vi "Facade 1.vi"(0 "Data In":T5, 2 "Display State In":T3, 3 "Container State":T4) -> (6 "Data Out":T5, 7 "Display State Out":T3, 8 "Action":T2)   [LabVIEW 2015, in "ECS-Host.lvlib" / "TrackingChart.xctl"]
uses:
  TrackingChart.xctl
  Data 1.ctl
  <vilib>/_xctls/Container State.ctl
  State 1.ctl
  <vilib>/_xctls/Action.ctl
  <vilib>/_xctls/XControlSupport.lvlib
panel:
  out "Chart":T1(graph)
  out "Indicator 1":sgl(slide) scale=0.0..25.0 scale format="%#.1f"
  out "Indicator 2":sgl(slide) scale=0.0..25.0 scale format="%#.1f"
  out "Indicator 3":sgl(slide) scale=0.0..25.0 scale format="%#.1f"
  out "Indicator 4":sgl(slide) scale=0.0..25.0 scale format="%#.1f"
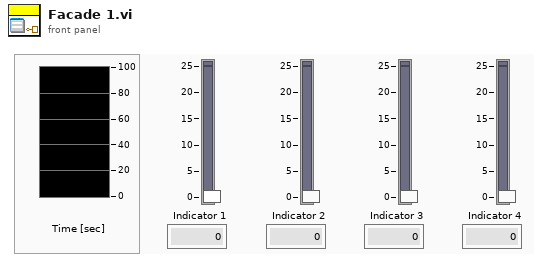
[diagram p1: front panel]
types:
  T1 = cluster{"[0]":sgl, "[1]":sgl, "[2]":sgl, "[3]":sgl, "[4]":sgl, "[5]":sgl, "[6]":sgl, "[7]":sgl, "[8]":sgl}
  T2 = typedef "XControlSupport.lvlib/Action.ctl" = cluster{"Data Changed?":bool, "State Changed?":bool, "Action Name":string}
  T3 = typedef "ECS-Host.lvlib/TrackingChart.xctl/State 1.ctl" = cluster{"Numeric":dbl}
  T4 = typedef "XControlSupport.lvlib/Container State.ctl" = cluster{"Indicator?":bool, "Run Mode?":bool, " Refnum":refnum<vi>}
  T5 = typedef "ECS-Host.lvlib/TrackingChart.xctl/Data 1.ctl" = cluster{"Value":sgl, "Name":string, "Unit":string, "Max":sgl, "Min":sgl}[]
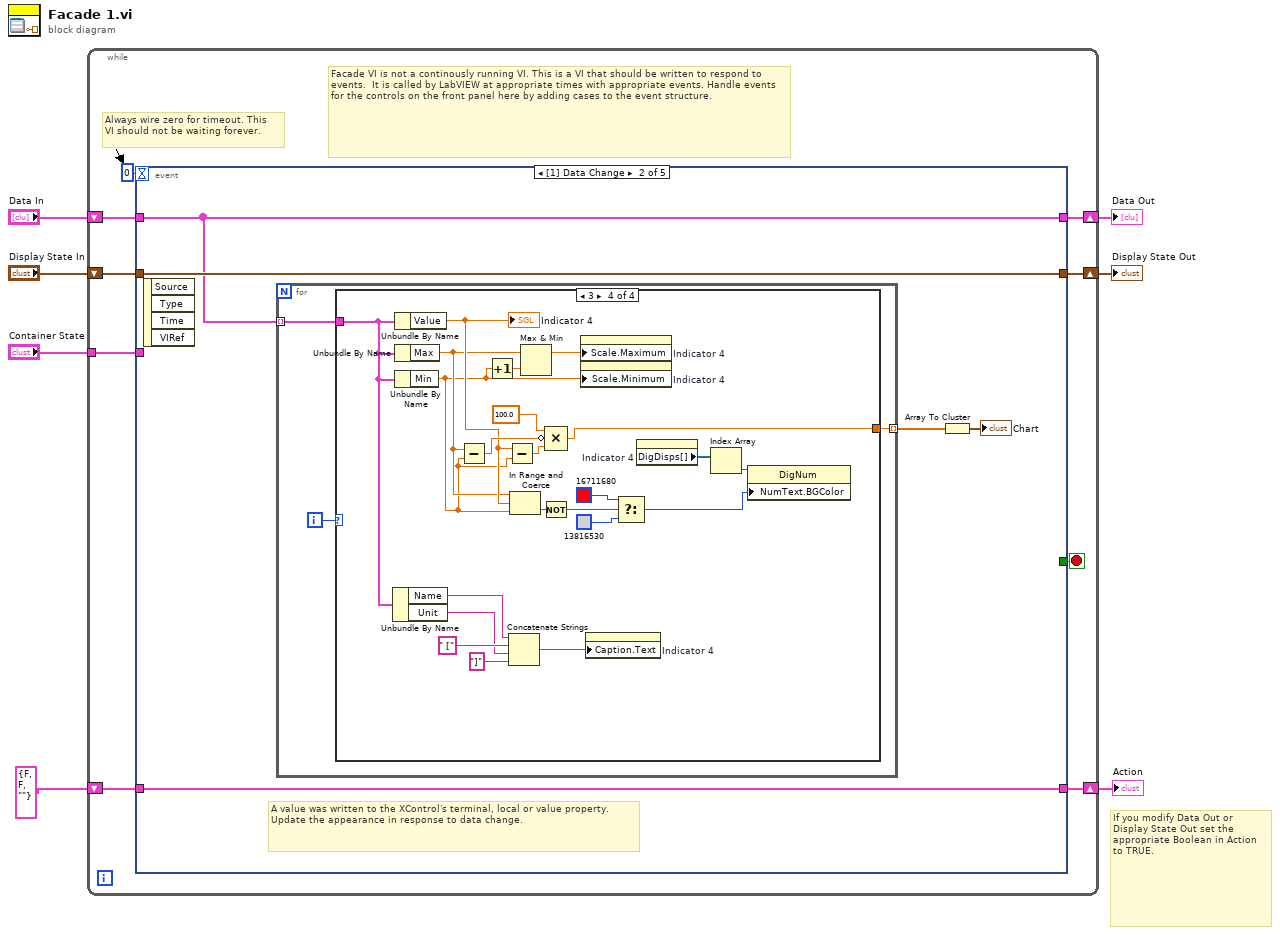
[diagram p0: block diagram]
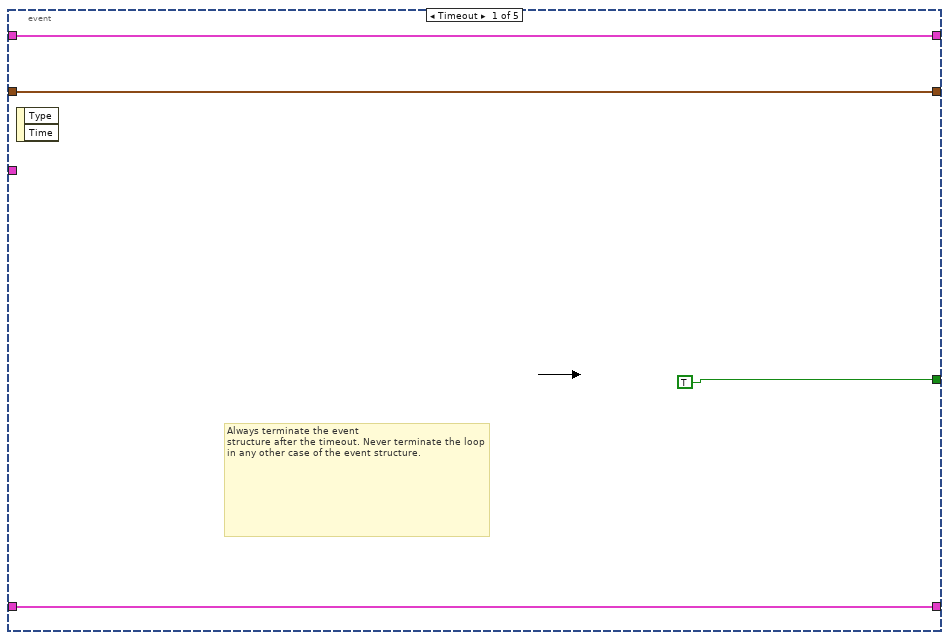
[diagram p2: hidden frame]
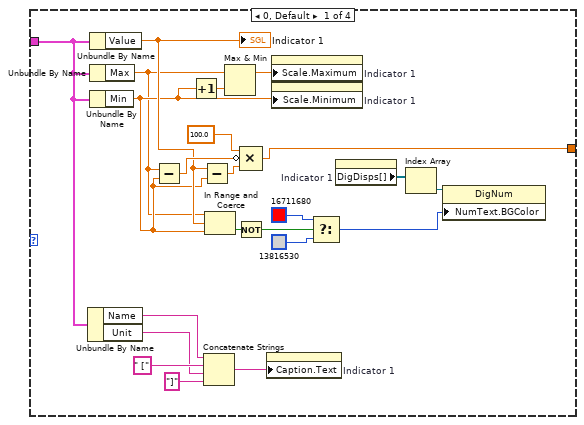
[diagram p3: hidden frame]
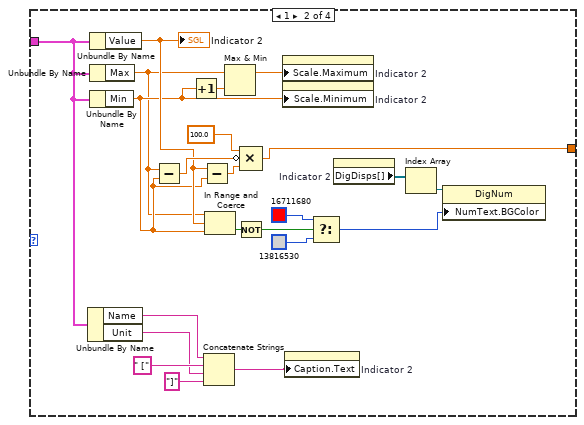
[diagram p4: hidden frame]
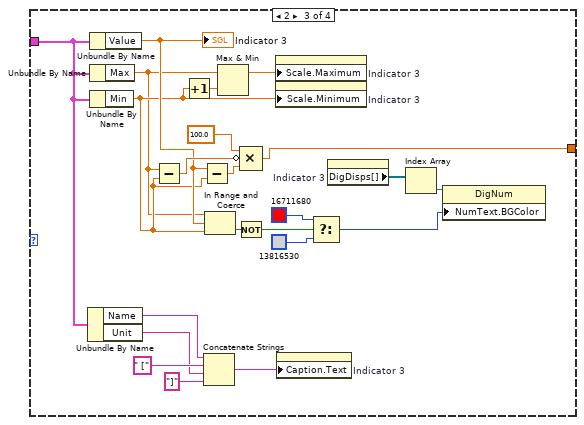
[diagram p5: hidden frame]
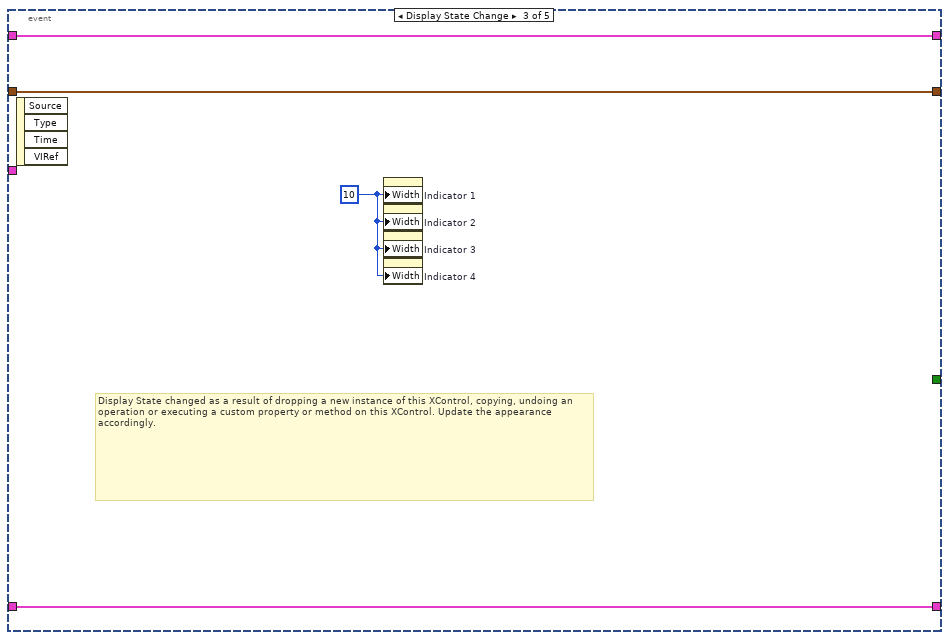
[diagram p6: hidden frame]
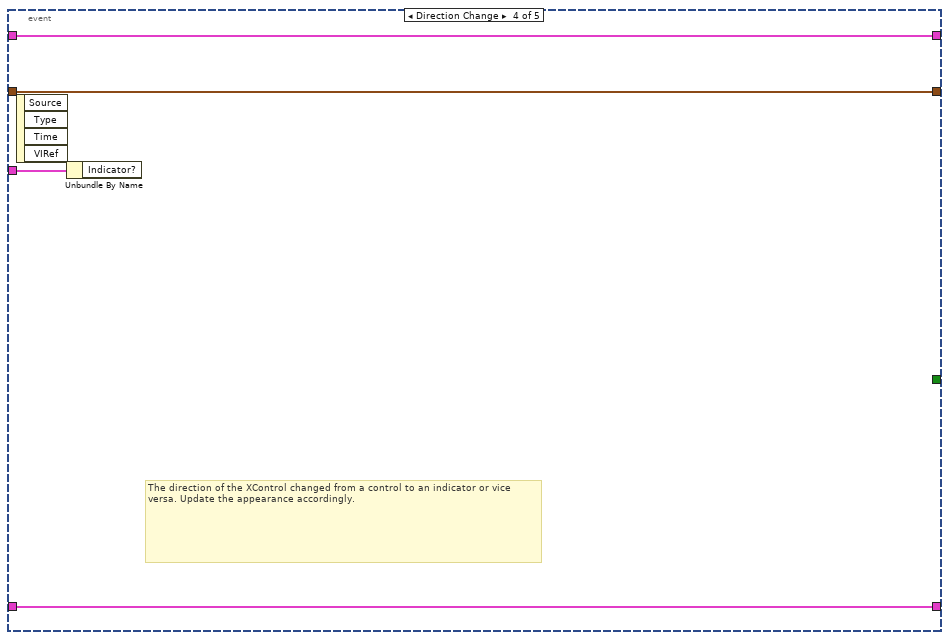
[diagram p7: hidden frame]
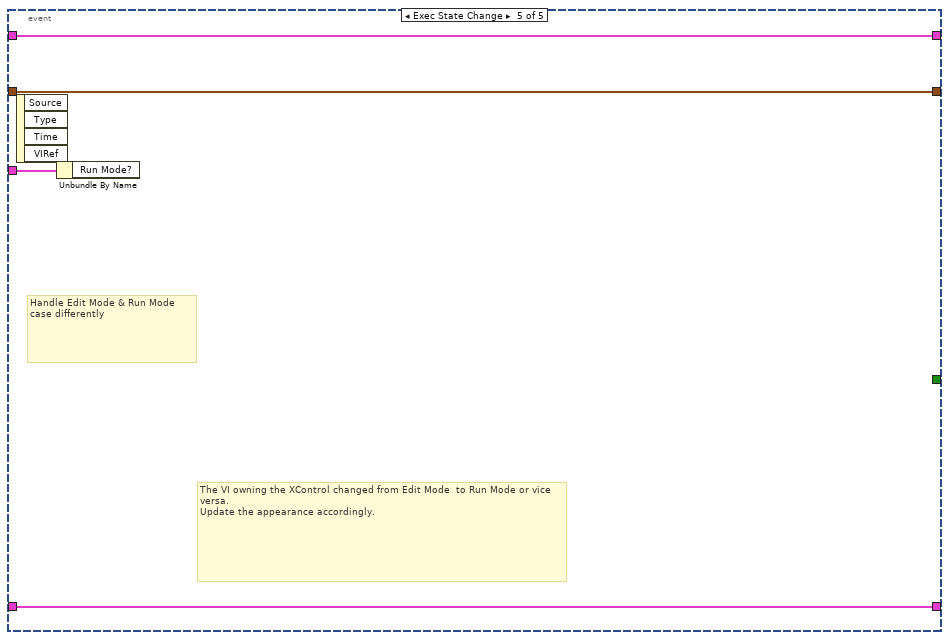
[diagram p8: hidden frame]
diagram:
  # "If you modify Data Out or\nDisplay State Out set the\nappropriate Boolean in Action\nto TRUE."
  n1 = while {
    shift-right: [w15] -> w4
    shift-left: "Display State In" -> [w16]
    tunnel: "Container State" -> [w12]
    shift-right: [w10] -> w7
    shift-left: "Data In" -> [w11]
    shift-right: [w8] -> w2
    shift-left: T2 {"Data Changed?"=FALSE, "State Changed?"=FALSE, "Action Name"=""} ("Action") -> [w9]
    stop <- w14 stop-if-true
    # "Facade VI is not a continously running VI. This is a VI that should be written to respond to events.  It is called by LabVIEW at appropriate times with appropriate events. Handle events for the controls on the front panel here by adding cases to the event structure."
    # "Always wire zero for timeout. This\nVI should not be waiting forever."
    n2 = event shown="[1] Data Change" {
      selector: _ -> [_ _ _ _ _]
      dyn-events: _ -> [_ _ _ _ _]
      timeout: 0 -> [_ _ _ _ _]
      tunnel: w16 -> [w18 w25 w120 w123 w127]
      tunnel: [w18 w25 w120 w123 w127] -> w15
      tunnel: [TRUE _ _ _ _] -> w14
      tunnel: w12 -> [_ _ _ w124 w128]
      tunnel: w11 -> [w17 w21 w118 w122 w125]
      tunnel: [w17 w21 w118 w122 w125] -> w10
      tunnel: [w19 w24 w119 w121 w126] -> w8
      tunnel: w9 -> [w19 w24 w119 w121 w126]
      event Timeout {
        # "Always terminate the event\nstructure after the timeout. Never terminate the loop in any other case of the event structure."
        n3 = event-data() -> ()  [unwired: 1 in, 2 out]
      }
      event Data Change {
        # "A value was written to the XControl's terminal, local or value property.\nUpdate the appearance in response to data change."
        n4 = event-data() -> ()  [unwired: 1 in, 4 out]
        n5 = for {
          tunnel: w21 -> [w27] mode=indexing
          tunnel: [w26] -> w22 mode=indexing
          i -> [w28]
          n6 = case shown="3" w28 {
            tunnel: w27 -> [w47 w69 w91 w113]
            tunnel: [w33 w58 w80 w102] -> w26
            frame 0, Default {
              n7 = Unbundle By Name(w47) -> ("Name"=w46:string, "Unit"=w48:string)
              n8 = Unbundle By Name(w47) -> ("Value"=w40:sgl)
              "Indicator 1" <- w40
              n9 = Unbundle By Name(w47) -> ("Max"=w29:sgl)
              n10 = Unbundle By Name(w47) -> ("Min"=w31:sgl)
              n11 = Subtract(x=w29, y=w31) -> (x-y=w42:sgl)
              n12 = Increment(x=w31) -> (x+1=w30:sgl)
              n13 = Subtract(x=w40, y=w31) -> (x-y=w44:sgl)
              n14 = Concatenate Strings(w46, " [", w48, "]") -> (w45:string)
              n15 = In Range and Coerce(upper limit=w29, x=w40, lower limit=w31) -> (In Range?=w41:bool)  [unwired: 1 out]
              n16 = Max & Min(x=w29, y=w30) -> (max(x,y)=w32:sgl)  [unwired: 1 out]
              n17 = Not(x=w41) -> (.not. x?=w37:bool)
              n18 = Compound Arithmetic op=MULTIPLY(sgl 100.0 ("value"), invert w42, w44) -> (w33:sgl)
              n19 = property on="Indicator 1" class="Slide (strict)"("Caption.Text"=w45) -> ()  [unwired: 2 in, 2 out]
              n20 = property on="Indicator 1" class="Slide (strict)"("Scale.Maximum"=w32) -> ()  [unwired: 2 in, 2 out]
              n21 = property on="Indicator 1" class="Slide (strict)"("Scale.Minimum"=w31) -> ()  [unwired: 2 in, 2 out]
              n22 = Select(t=u32 16711680, s=w37, f=u32 13816530) -> (s? t:f=w36:u32)
              n23 = property on="Indicator 1" class="Slide (strict)"() -> ("DigDisps[]"=w35:refnum<vi>[])  [unwired: 2 in, 2 out]
              n24 = Index Array(array=w35) -> (element=w34:refnum<vi>)  [unwired: 1 in]
              n25 = property class="DigNum"(reference=w34, "NumText.BGColor"=w36) -> ()  [unwired: 1 in, 2 out]
            }
            frame 1 {
              n26 = Unbundle By Name(w69) -> ("Name"=w68:string, "Unit"=w70:string)
              n27 = Unbundle By Name(w69) -> ("Value"=w55:sgl)
              "Indicator 2" <- w55
              n28 = Unbundle By Name(w69) -> ("Max"=w51:sgl)
              n29 = Unbundle By Name(w69) -> ("Min"=w53:sgl)
              n30 = Subtract(x=w51, y=w53) -> (x-y=w65:sgl)
              n31 = Increment(x=w53) -> (x+1=w54:sgl)
              n32 = Subtract(x=w55, y=w53) -> (x-y=w67:sgl)
              n33 = Concatenate Strings(w68, " [", w70, "]") -> (w57:string)
              n34 = In Range and Coerce(upper limit=w51, x=w55, lower limit=w53) -> (In Range?=w64:bool)  [unwired: 1 out]
              n35 = Max & Min(x=w51, y=w54) -> (max(x,y)=w52:sgl)  [unwired: 1 out]
              n36 = Not(x=w64) -> (.not. x?=w61:bool)
              n37 = Compound Arithmetic op=MULTIPLY(sgl 100.0 ("value"), invert w65, w67) -> (w58:sgl)
              n38 = property on="Indicator 2" class="Slide (strict)"("Scale.Maximum"=w52) -> ()  [unwired: 2 in, 2 out]
              n39 = property on="Indicator 2" class="Slide (strict)"("Scale.Minimum"=w53) -> ()  [unwired: 2 in, 2 out]
              n40 = property on="Indicator 2" class="Slide (strict)"("Caption.Text"=w57) -> ()  [unwired: 2 in, 2 out]
              n41 = Select(t=u32 16711680, s=w61, f=u32 13816530) -> (s? t:f=w60:u32)
              n42 = property on="Indicator 2" class="Slide (strict)"() -> ("DigDisps[]"=w56:refnum<vi>[])  [unwired: 2 in, 2 out]
              n43 = Index Array(array=w56) -> (element=w59:refnum<vi>)  [unwired: 1 in]
              n44 = property class="DigNum"(reference=w59, "NumText.BGColor"=w60) -> ()  [unwired: 1 in, 2 out]
            }
            frame 2 {
              n45 = Unbundle By Name(w91) -> ("Name"=w90:string, "Unit"=w92:string)
              n46 = Unbundle By Name(w91) -> ("Value"=w79:sgl)
              "Indicator 3" <- w79
              n47 = Unbundle By Name(w91) -> ("Max"=w73:sgl)
              n48 = Unbundle By Name(w91) -> ("Min"=w75:sgl)
              n49 = Subtract(x=w73, y=w75) -> (x-y=w87:sgl)
              n50 = Increment(x=w75) -> (x+1=w76:sgl)
              n51 = Subtract(x=w79, y=w75) -> (x-y=w89:sgl)
              n52 = Concatenate Strings(w90, " [", w92, "]") -> (w78:string)
              n53 = In Range and Coerce(upper limit=w73, x=w79, lower limit=w75) -> (In Range?=w86:bool)  [unwired: 1 out]
              n54 = Max & Min(x=w73, y=w76) -> (max(x,y)=w74:sgl)  [unwired: 1 out]
              n55 = Not(x=w86) -> (.not. x?=w83:bool)
              n56 = Compound Arithmetic op=MULTIPLY(sgl 100.0 ("value"), invert w87, w89) -> (w80:sgl)
              n57 = property on="Indicator 3" class="Slide (strict)"("Scale.Maximum"=w74) -> ()  [unwired: 2 in, 2 out]
              n58 = property on="Indicator 3" class="Slide (strict)"("Scale.Minimum"=w75) -> ()  [unwired: 2 in, 2 out]
              n59 = property on="Indicator 3" class="Slide (strict)"("Caption.Text"=w78) -> ()  [unwired: 2 in, 2 out]
              n60 = Select(t=u32 16711680, s=w83, f=u32 13816530) -> (s? t:f=w82:u32)
              n61 = property on="Indicator 3" class="Slide (strict)"() -> ("DigDisps[]"=w77:refnum<vi>[])  [unwired: 2 in, 2 out]
              n62 = Index Array(array=w77) -> (element=w81:refnum<vi>)  [unwired: 1 in]
              n63 = property class="DigNum"(reference=w81, "NumText.BGColor"=w82) -> ()  [unwired: 1 in, 2 out]
            }
            frame 3 {
              n64 = Unbundle By Name(w113) -> ("Name"=w112:string, "Unit"=w114:string)
              n65 = Unbundle By Name(w113) -> ("Value"=w100:sgl)
              "Indicator 4" <- w100
              n66 = Unbundle By Name(w113) -> ("Max"=w96:sgl)
              n67 = Unbundle By Name(w113) -> ("Min"=w95:sgl)
              n68 = Subtract(x=w96, y=w95) -> (x-y=w109:sgl)
              n69 = Increment(x=w95) -> (x+1=w97:sgl)
              n70 = Subtract(x=w100, y=w95) -> (x-y=w111:sgl)
              n71 = Concatenate Strings(w112, " [", w114, "]") -> (w101:string)
              n72 = In Range and Coerce(upper limit=w96, x=w100, lower limit=w95) -> (In Range?=w108:bool)  [unwired: 1 out]
              n73 = Max & Min(x=w96, y=w97) -> (max(x,y)=w98:sgl)  [unwired: 1 out]
              n74 = Not(x=w108) -> (.not. x?=w105:bool)
              n75 = Compound Arithmetic op=MULTIPLY(sgl 100.0 ("value"), invert w109, w111) -> (w102:sgl)
              n76 = property on="Indicator 4" class="Slide (strict)"("Scale.Maximum"=w98) -> ()  [unwired: 2 in, 2 out]
              n77 = property on="Indicator 4" class="Slide (strict)"("Scale.Minimum"=w95) -> ()  [unwired: 2 in, 2 out]
              n78 = property on="Indicator 4" class="Slide (strict)"("Caption.Text"=w101) -> ()  [unwired: 2 in, 2 out]
              n79 = Select(t=u32 16711680, s=w105, f=u32 13816530) -> (s? t:f=w104:u32)
              n80 = property on="Indicator 4" class="Slide (strict)"() -> ("DigDisps[]"=w99:refnum<vi>[])  [unwired: 2 in, 2 out]
              n81 = Index Array(array=w99) -> (element=w103:refnum<vi>)  [unwired: 1 in]
              n82 = property class="DigNum"(reference=w103, "NumText.BGColor"=w104) -> ()  [unwired: 1 in, 2 out]
            }
          }
        }
        n83 = Array To Cluster(array=w22) -> (cluster=→"Chart":T1)
      }
      event Display State Change {
        w117 = u32 10 ("Housing Size:Width")
        # "Display State changed as a result of dropping a new instance of this XControl, copying, undoing an operation or executing a custom property or method on this XControl. Update the appearance accordingly."
        n84 = event-data() -> ()  [unwired: 1 in, 4 out]
        n85 = property on="Indicator 1" class="Slide (strict)"("Width"=w117) -> ()  [unwired: 2 in, 2 out]
        n86 = property on="Indicator 2" class="Slide (strict)"("Width"=w117) -> ()  [unwired: 2 in, 2 out]
        n87 = property on="Indicator 3" class="Slide (strict)"("Width"=w117) -> ()  [unwired: 2 in, 2 out]
        n88 = property on="Indicator 4" class="Slide (strict)"("Width"=w117) -> ()  [unwired: 2 in, 2 out]
      }
      event Direction Change {
        # "The direction of the XControl changed from a control to an indicator or vice versa. Update the appearance accordingly."
        n89 = event-data() -> ()  [unwired: 1 in, 4 out]
        n90 = Unbundle By Name(w124) -> ()  [unwired: 1 out]
      }
      event Exec State Change {
        # "The VI owning the XControl changed from Edit Mode  to Run Mode or vice versa.\nUpdate the appearance accordingly."
        # "Handle Edit Mode & Run Mode\ncase differently"
        n91 = event-data() -> ()  [unwired: 1 in, 4 out]
        n92 = Unbundle By Name(w128) -> ()  [unwired: 1 out]
      }
    }
  }
  "Display State Out" <- w4
  "Data Out" <- w7
  "Action" <- w2
